vi "about.vi"   [LabVIEW 2016]
panel:
  # "Software Versão 1.0.2017               Lucasoliveira@globomail.com"
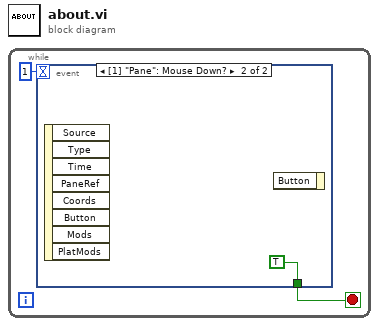
[diagram p0: block diagram]
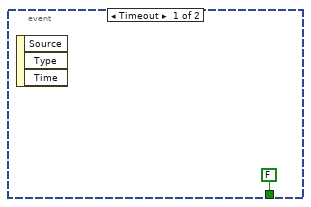
[diagram p2: hidden frame]
diagram:
  n1 = while {
    stop <- w2 stop-if-true
    n2 = event shown="[1] \"Pane\": Mouse Down?" {
      selector: _ -> [_ _]
      dyn-events: _ -> [_ _]
      timeout: 1 -> [_ _]
      tunnel: [FALSE TRUE] -> w2
      event Timeout {
        n3 = event-data() -> ()  [unwired: 1 in, 3 out]
      }
      event Mouse Down? {
        n4 = event-data() -> ()  [unwired: 1 in, 8 out]
        n5 = event-data() -> ()  [unwired: 2 in, 1 out]
      }
    }
  }
